vi "RT Obtain Notifier.vi"(7 "Case":enum16{"Obtain", "Read"}(ring), 8 "error in (no error)":errorcluster) -> (0 "error out":errorcluster, 3 "All Notifier":T1)   [LabVIEW 2022 SP3]
uses:
  RT Controls/RT All Notifer.ctl
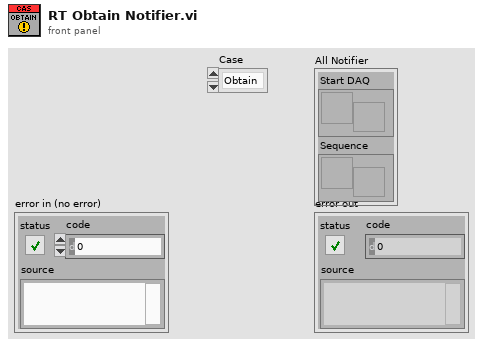
[diagram p1: front panel]
types:
  T1 = typedef "RT All Notifer.ctl" = cluster{"Start DAQ":refnum<notifier>, "Sequence":refnum<notifier>}
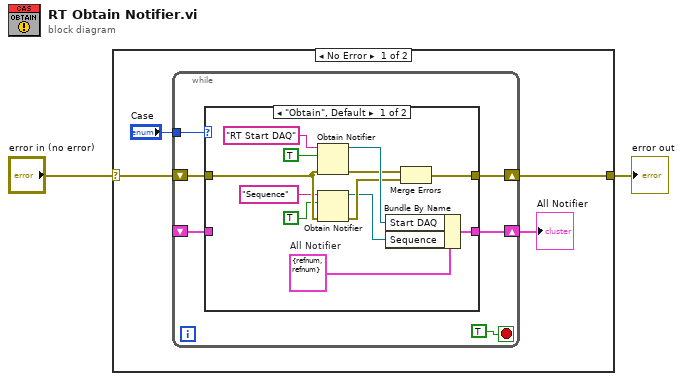
[diagram p0: block diagram]
diagram:
  n1 = case shown="No Error" "error in (no error)" {
    selector: "error in (no error)" -> [w6 w27]
    tunnel: [w5 w27] -> w1
    frame No Error {
      n2 = while {
        shift-right: [w11] -> w5
        shift-left: w6 -> [w12]
        tunnel: "Case" -> [w9]
        shift-right: [w8] -> w3
        shift-left: _ -> [w7]
        stop <- TRUE stop-if-true
        n3 = case shown="\"Obtain\", Default" w9 {
          tunnel: w12 -> [w19 w25]
          tunnel: [w18 w25] -> w11
          tunnel: [w22 w26] -> w8
          tunnel: w7 -> [_ w26]
          frame "Obtain", Default {
            w24 = T1 {"Start DAQ"=refnum, "Sequence"=refnum}  # All Notifier
            n4 = Obtain Notifier(name (unnamed)="RT Start DAQ", notification data type=TRUE ("create if not found? (T)"), error in (no error)=w19) -> (notifier out=w20:refnum<notifier>, error out=w17:errorcluster)  [unwired: 1 in, 1 out]
            n5 = Obtain Notifier(name (unnamed)="Sequence", notification data type=TRUE ("create if not found? (T)"), error in (no error)=w19) -> (notifier out=w13:refnum<notifier>, error out=w16:errorcluster)  [unwired: 1 in, 1 out]
            n6 = Bundle By Name(cluster=w24, "Start DAQ"=w20, "Sequence"=w13) -> (w22:T1)
            n7 = Merge Errors(w17, w16) -> (w18:errorcluster)
          }
          frame "Read" {
          }
        }
      }
      "All Notifier" <- w3
    }
    frame Error {
    }
  }
  "error out" <- w1
